vi "Labspec Acquire.vi"(0 "Automation Refnum In":refnum<k7>, 1 "From (nm)":dbl=1.0, 2 "To (nm)":dbl=1.0, 5 "Mode":T3 items=["Spectrum", "Image", "Spectrum (Labspec Parameters)", "Spectral Image", "Get Detector Temperature", "Real Time Acquisition", "Set Photomultiplier Parameter", "Macro Spot", "Cancel Acquisition", "Set Detector"], 7 "Shutter Mode":T2 items=[" "=0, "Auto Scanning"=1000, "Don't Close Shutter"=2000, "Accumulation Mode"=10000], 9 "Data Treatment":T1 items=[" "=0, "Auto Show"=10, "No Spike Removing"=100, "Single Spike Removing"=200, "Double Spike Removing"=300, "Double Spike Removing with Autoadd"=400], 11 "error in":errorcluster, 12 "Number of Accumulations":i32, 13 "Integration Time (s)":dbl=1.0) -> (4 "Automation Refnum Out":refnum<k7>, 6 "Acq":i32, 8 "AcqID":i32, 15 "error out":errorcluster)   [LabVIEW 2014]
uses:
  Acquire Mode.ctl
  Acquire Shutter Mode.ctl
  Acquire Data Handling.ctl
panel:
  # "LICENSED MATERIALS – PROPERTY OF IBM\nCopyright IBM Corp. 2016,\nALL RIGHTS RESERVED"
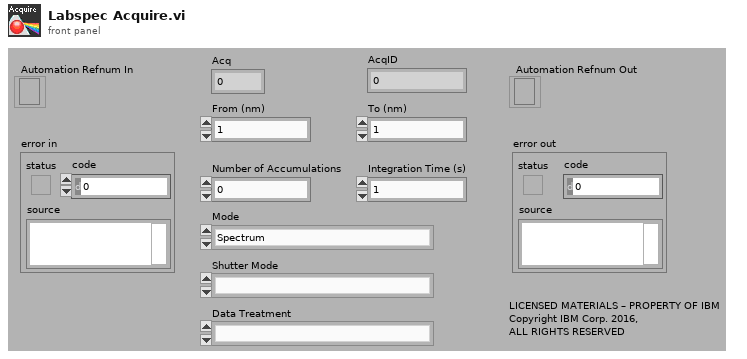
[diagram p1: front panel]
types:
  T1 = typedef "Acquire Data Handling.ctl" = u16
  T2 = typedef "Acquire Shutter Mode.ctl" = u16
  T3 = typedef "Acquire Mode.ctl" = u16
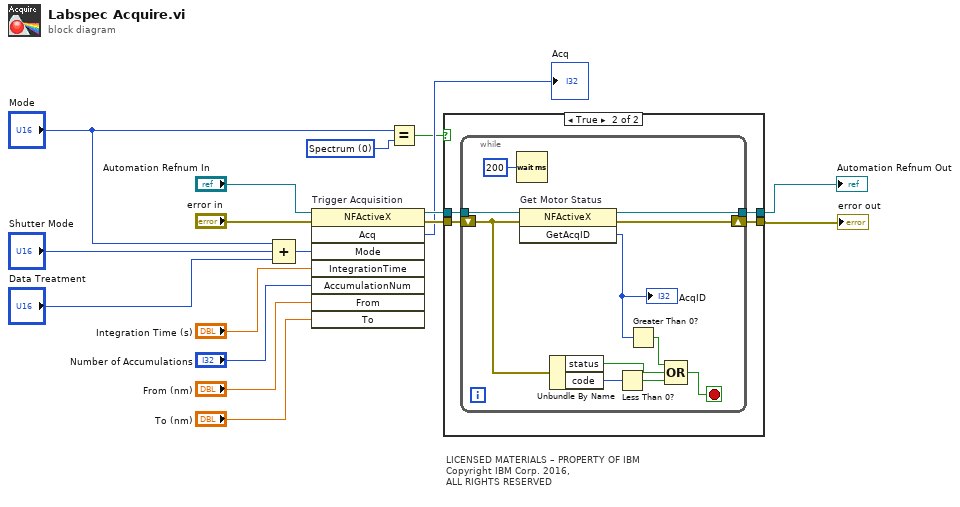
[diagram p0: block diagram]
diagram:
  w3 = T3 0 items=["Spectrum", "Image", "Spectrum (Labspec Parameters)", "Spectral Image", "Get Detector Temperature", "Real Time Acquisition", "Set Photomultiplier Parameter", "Macro Spot", "Cancel Acquisition", "Set Detector"] ("Mode")
  # "LICENSED MATERIALS – PROPERTY OF IBM\nCopyright IBM Corp. 2016,\nALL RIGHTS RESERVED"
  n1 = Compound Arithmetic op=ADD("Mode", "Shutter Mode", "Data Treatment") -> (w9:T3)
  n2 = invoke on="Trigger Acquisition" class="NFActiveX" method="Acq"(reference="Automation Refnum In", error in="error in", "Mode"=w9, "IntegrationTime"="Integration Time (s)", "AccumulationNum"="Number of Accumulations", "From"="From (nm)", "To"="To (nm)") -> (reference out=w13:refnum<k7>, error out=w12:errorcluster, "Acq"=→"Acq":i32)  [unwired: 1 in, 5 out]
  n3 = Equal?(x="Mode", y=w3) -> (x = y?=w4:bool)
  n4 = case shown="True" w4 {
    tunnel: w13 -> [w19 w23]
    tunnel: w12 -> [w18 w22]
    tunnel: [w18 w21] -> w2
    tunnel: [w19 w20] -> w10
    frame False {
    }
    frame True {
      n5 = while {
        tunnel: w23 -> [w33]
        tunnel: [w32] -> w20
        shift-right: [w31] -> w21
        shift-left: w22 -> [w27]
        stop <- w25 stop-if-true
        n6 = Wait (ms)(milliseconds to wait=u32 200) -> ()  [unwired: 1 out]
        n7 = invoke on="Get Motor Status" class="NFActiveX" method="GetAcqID"(reference=w33, error in=w27) -> (reference out=w32:refnum<k7>, error out=w31:errorcluster, "GetAcqID"=w24:i32)  [unwired: 1 in]
        "AcqID" <- w24
        n8 = Unbundle By Name(w27) -> ("status"=w29:bool, "code"=w30:i32)
        n9 = Less Than 0?(x=w30) -> (x < 0?=w28:bool)
        n10 = Greater Than 0?(x=w24) -> (x > 0?=w26:bool)
        n11 = Compound Arithmetic op=OR(w26, w29, w28) -> (w25:bool)
      }
    }
  }
  "error out" <- w2
  "Automation Refnum Out" <- w10
